vi "Module To Position Lookup.vi"(10 "NewSetup":T2) -> (1 "TR Module/Raster num":i32, 2 "Position":T1, 4 "Polarization":u16(ring) items=["Horizontal", "Vertical"])   [LabVIEW 2017]
doc: "for now Modules are enumerated 0 - 15,\nPositions 1 - 16"
uses:
  Classes/Sequence/SequenceSubvis/RF Direction.ctl
  Classes/Sequence/SequenceSubvis/PolarizationSelect.ctl
  Classes/Sequence/SequenceSubvis/PatchNewTestStep.ctl
  VXM Public API/mmWaveAxis.ctl
  VXM Public API/singleAxisMoveDef.ctl
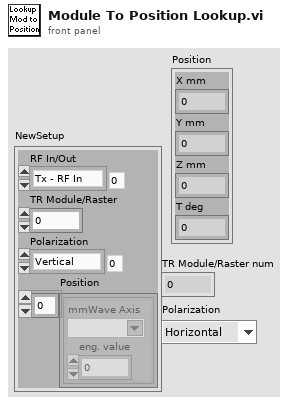
[diagram p1: front panel]
types:
  T1 = cluster{"X mm":dbl, "Y mm":dbl, "Z mm":dbl, "T deg":dbl}
  T2 = typedef "PatchNewTestStep.ctl" = cluster{"RF In/Out":T3, "TR Module/Raster":i32, "Polarization":T4, "Position":T5[]}
  T3 = typedef "RF Direction.ctl" = enum16{"Tx - RF In", "Rx - RF Out"}
  T4 = typedef "PolarizationSelect.ctl" = enum16{"Vertical", "Horizontal"}
  T5 = typedef "singleAxisMoveDef.ctl" = cluster{"mmWave Axis":T6, "eng. value":dbl}
  T6 = typedef "mmWaveAxis.ctl" = string
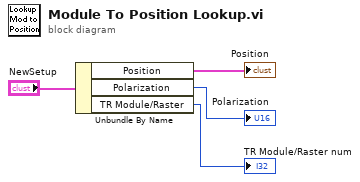
[diagram p0: block diagram]
diagram:
  n1 = Unbundle By Name("NewSetup") -> ("Position"=→"Position":T5[], "Polarization"=→"Polarization":T4, "TR Module/Raster"=→"TR Module/Raster num":i32)
